vi "GetFrontPanel.vi"(8 "ErrorIn":errorcluster, 11 "ObjectIn":refnum<class "IFrontPanel.lvclass">) -> (0 "ErrorOut":errorcluster, 2 "FrontPanelControl":refnum<class "FrontPanelControl.lvclass">, 3 "ObjectOut":refnum<class "IFrontPanel.lvclass">)   [LabVIEW 2021, in "IFrontPanel.lvclass"]
uses:
  IFrontPanel.lvclass
  Library_UserInterface_FrontPanelControl/FrontPanelControl/FrontPanelControl.lvclass
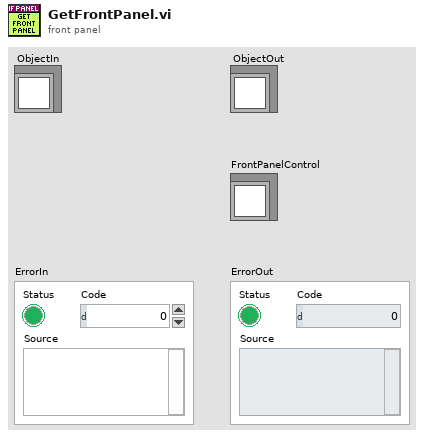
[diagram p1: front panel]
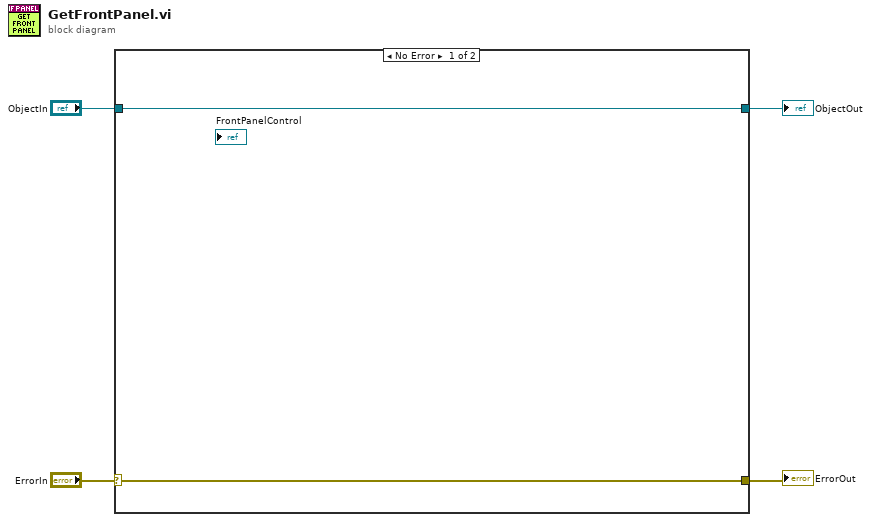
[diagram p0: block diagram]
diagram:
  n1 = case shown="No Error" "ErrorIn" {
    selector: "ErrorIn" -> [w6 w8]
    tunnel: [w6 w8] -> w3
    tunnel: [w5 w7] -> w1
    tunnel: "ObjectIn" -> [w5 w7]
    frame No Error {
    }
    frame Error {
    }
  }
  "ErrorOut" <- w3
  "ObjectOut" <- w1
